vi "CheckTiming.vi"(8 "error in (no error)":errorcluster, 10 "Message Queues":T3, 11 "MessageSetList":T1) -> (0 "error out":errorcluster, 3 "Array":T2[](array[typedef]))   [LabVIEW 2017, in "Server.lvlib" / "Timing.lvlib"]
doc: "Iterates though all Timing Sets and checks, if the Time has expired for this specific Set. If yes, it sends the Message to MHL."
uses:
  Timing.lvlib
  Message Queue/CommReferences.ctl
  Message Queue/MessageCluster.ctl
  MessageSet.ctl
  MessageSetList.ctl
  Message Queue/EnqueueMessage(Single).vi
  Message Queue/Message Queue.lvlib
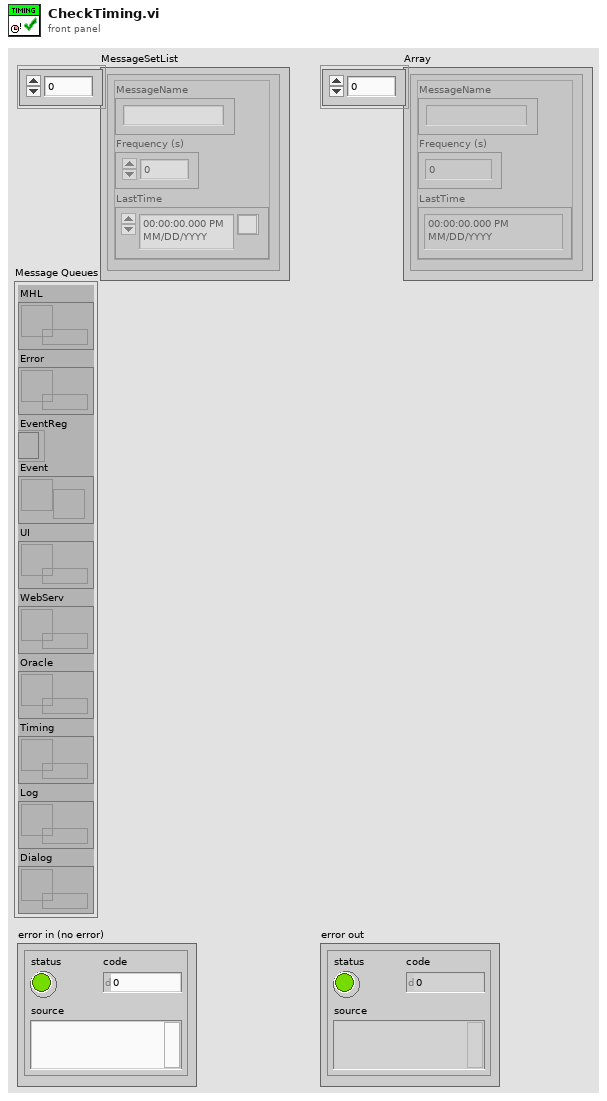
[diagram p1: front panel]
types:
  T1 = typedef "Server.lvlib/Timing.lvlib/MessageSetList.ctl" = T2[]
  T2 = typedef "Server.lvlib/Timing.lvlib/MessageSet.ctl" = cluster{"MessageName":string, "Frequency (s)":dbl, "LastTime":timestamp}
  T3 = typedef "Server.lvlib/Message Queue.lvlib/CommReferences.ctl" = cluster{"MHL":refnum<queue>, "Error":refnum<queue>, "EventReg":refnum<event-registration>, "Event":refnum<user-event>, "UI":refnum<queue>, "WebServ":refnum<queue>, "Oracle":refnum<queue>, "Timing":refnum<queue>, "Log":refnum<queue>, "Dialog":refnum<queue>}
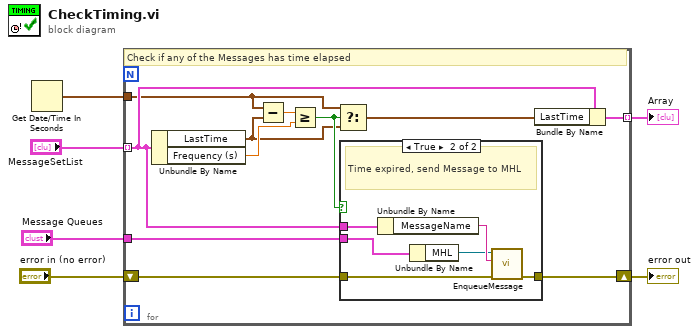
[diagram p0: block diagram]
diagram:
  n1 = Get Date/Time In Seconds() -> (seconds since 1Jan1904=w2:timestamp)
  n2 = for {
    tunnel: "MessageSetList" -> [w12] mode=indexing
    tunnel: w2 -> [w8]
    tunnel: [w15] -> w3 mode=indexing
    shift-right: [w14] -> w6
    shift-left: "error in (no error)" -> [w13]
    tunnel: "Message Queues" -> [w11]
    # "Check if any of the Messages has time elapsed"
    n3 = Unbundle By Name(w12) -> ("LastTime"=w9:timestamp, "Frequency (s)"=w16:dbl)
    n4 = Subtract(x=w8, y=w9) -> (x-y=w17:dbl)
    n5 = Greater Or Equal?(x=w17, y=w16) -> (x >= y?=w10:bool)
    n6 = Select(t=w8, s=w10, f=w9) -> (s? t:f=w7:timestamp)
    n7 = case shown="True" w10 {
      tunnel: [w18 w23] -> w14
      tunnel: w13 -> [w18 w24]
      tunnel: w12 -> [_ w22]
      tunnel: w11 -> [_ w20]
      frame False {
      }
      frame True {
        # "Time expired, send Message to MHL"
        n8 = Unbundle By Name(w22) -> ("MessageName"=w21:string)
        n9 = Unbundle By Name(w20) -> ("MHL"=w19:refnum<queue>)
        n10 = call-poly "EnqueueMessage.vi"("error in (no error)"=w24, "Message"=w21, "Message Queue"=w19) -> ("error out"=w23:errorcluster)  [unwired: 7 in, 1 out]
      }
    }
    n11 = Bundle By Name(cluster=w12, "LastTime"=w7) -> (w15:T2)
  }
  "error out" <- w6
  "Array" <- w3
